vi "TDS Comms Write Data.vi"(8 "error in (no error)":errorcluster, 9 "Write Settings":string, 10 "Write Data":string, 11 "Address":string) -> (0 "error out":errorcluster, 3 "Actual Write Data":string)   [LabVIEW 2025, in "Interface Functions.lvlib"]
uses:
  Interface Functions.lvlib
  <vilib>/Utility/error.llb/Trim Whitespace One-Sided.vi
  <vilib>/Utility/error.llb/Error Cluster From Error Code.vi
  <vilib>/ErrorRing/Error Ring.xnode
panel:
  out "Read Data":string
  out "standard error":string
  # "Comms Write Data"
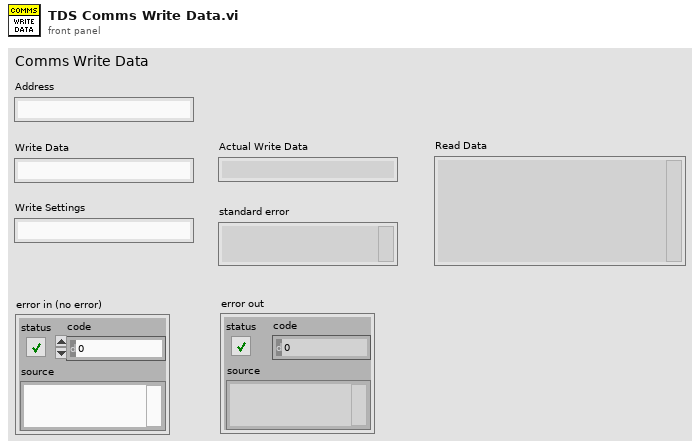
[diagram p1: front panel]
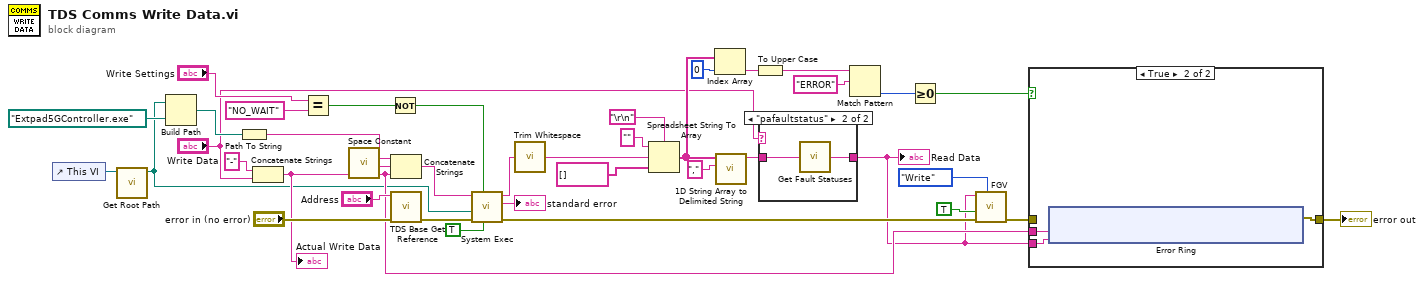
[diagram p0: block diagram]
diagram:
  n1 = control-ref of="This VI"() -> (w5:refnum<vi>)
  n2 = call "Get Root Path.vi"("VI in"=w5) -> ("Extpad Directory"=w4:path)  [unwired: 10 in]
  n3 = Build Path(base path=w4, name or relative path=path "Extpad5GController.exe") -> (appended path=w35:path)
  n4 = Path To String(path=w35) -> (string=w32:string)
  n5 = Concatenate Strings("-" ("string"), "Write Data") -> (w14:string)
  "Actual Write Data" <- w14
  n6 = Equal?(x="Write Settings", y="NO_WAIT") -> (x = y?=w11:bool)
  n7 = call <vilib>:"Space Constant.vi"() -> ("String"=w31:string)
  n8 = Not(x=w11) -> (.not. x?=w10:bool)
  n9 = Concatenate Strings(w32, w31, w14) -> (w30:string)
  n10 = call "TDS Base Get Reference.vi"("error in (no error)"="error in (no error)", "Address"="Address") -> ("error out"=w34:errorcluster)  [unwired: 8 in, 1 out]
  n11 = call <vilib>:"System Exec.vi"("run minimized? (F)"=TRUE, "wait until completion? (T)"=w10, "error in (no error)"=w34, "working directory"=w4, "command line"=w30) -> ("error out"=w9:errorcluster, "standard error"=→"standard error":string, "standard output"=w26:string)  [unwired: 3 in, 1 out]
  n12 = call <vilib>:"Trim Whitespace.vi"("string"=w26) -> ("trimmed string"=w27:string)  [unwired: 1 in]
  n13 = Spreadsheet String To Array(delimiter (Tab)="\r\n", format string="", spreadsheet string=w27, array type (2D Dbl)=string[] []) -> (array=w16:string[])
  n14 = Index Array(array=w16, index=0) -> (element=w22:string)
  n15 = call <vilib>:"1D String Array to Delimited String.vi"("delimiter"=",", "string array"=w16) -> ("delimited string"=w2:string)  [unwired: 9 in]
  n16 = To Upper Case(1:w22) -> (0:w21:string)
  n17 = case shown="\"pafaultstatus\"" "Write Data" {
    tunnel: w2 -> [w40 w42]
    tunnel: [w40 w41] -> w1
    frame Default {
    }
    frame "pafaultstatus" {
      n18 = call "Get Fault Statuses.vi"("Fault String"=w42) -> ("Fault Descriptions"=w41:string)  [unwired: 4 in]
    }
  }
  "Read Data" <- w1
  n19 = Match Pattern(string=w21, regular expression="ERROR") -> (offset past match=w19:i32)  [unwired: 1 in, 3 out]
  n20 = Greater Or Equal To 0?(x=w19) -> (x >= 0?=w18:bool)
  n21 = call "FGV.vi"("Action"=enum16{"Initialize", "Read", "Write"}."Write", "error in (no error)"=w9, "Successful"=TRUE, "Read Data"=w1) -> ("error out"=w7:errorcluster)  [unwired: 5 in, 2 out]
  n22 = case shown="True" w18 {
    tunnel: w7 -> [w43 _]
    tunnel: [w43 w46] -> w17
    tunnel: w1 -> [_ w45]
    tunnel: w14 -> [_ w44]
    frame False {
    }
    frame True {
      n23 = xnode "Error Ring"("parameter 0"=w44, "parameter 1"=w45) -> ("error out"=w46:errorcluster)
    }
  }
  "error out" <- w17
